vi "실습 5-4 열거형 케이스 선택자.vi"() -> ()   [LabVIEW 2014]
uses:
  <vilib>/measure/NI_MABase.lvlib
panel:
  in  "정지":bool
  in  "열거형":enum16{"사인파", "삼각파", "톱니파", "DC 신호", "노이즈"}(ring)=enum."톱니파"
  out "웨이브폼 그래프":waveform(dbl)(graph)
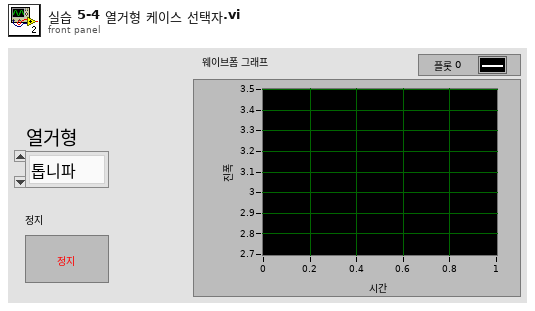
[diagram p1: front panel]
types:
  T1 = enum16{"Sine Wave", "Triangle Wave", "Square Wave", "Sawtooth Wave"}
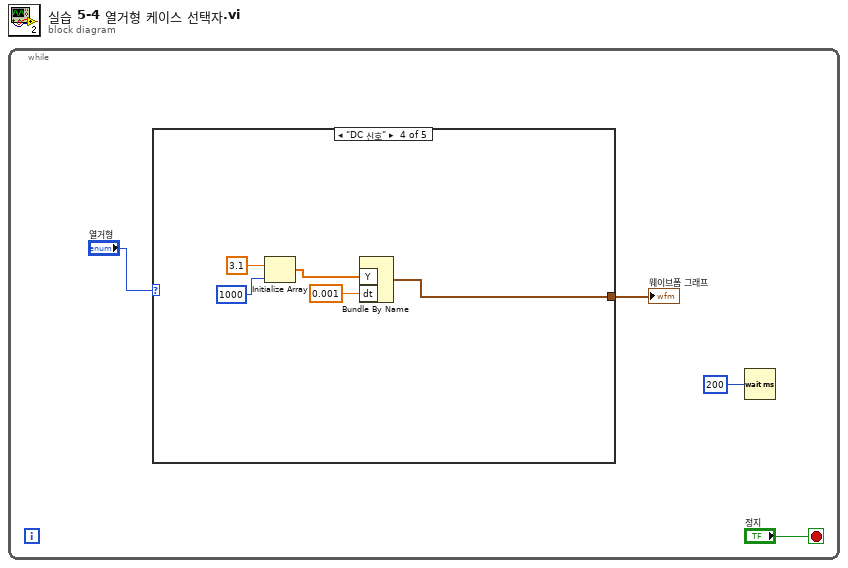
[diagram p0: block diagram]
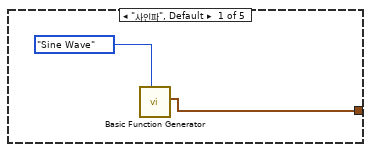
[diagram p2: hidden frame]
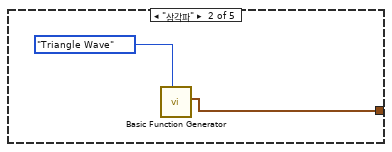
[diagram p3: hidden frame]
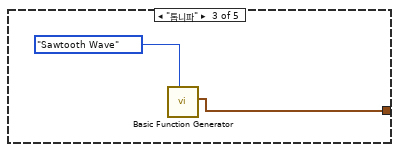
[diagram p4: hidden frame]
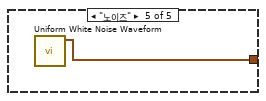
[diagram p5: hidden frame]
diagram:
  n1 = while {
    stop <- "정지" stop-if-true
    n2 = case shown="\"DC 신호\"" "열거형" {
      tunnel: [w5 w7 w9 w12 w16] -> w3
      frame "사인파", Default {
        n3 = call <vilib>:"Basic Function Generator.vi"("signal type"=T1."Sine Wave") -> ("signal out"=w5:waveform(dbl))  [unwired: 8 in, 2 out]
      }
      frame "삼각파" {
        n4 = call <vilib>:"Basic Function Generator.vi"("signal type"=T1."Triangle Wave") -> ("signal out"=w7:waveform(dbl))  [unwired: 8 in, 2 out]
      }
      frame "톱니파" {
        n5 = call <vilib>:"Basic Function Generator.vi"("signal type"=T1."Sawtooth Wave") -> ("signal out"=w9:waveform(dbl))  [unwired: 8 in, 2 out]
      }
      frame "DC 신호" {
        n6 = Initialize Array(3.1 ("원소"), 1000 ("차원 크기")) -> (w13:dbl[])
        n7 = Bundle By Name("Y"=w13, "dt"=0.001) -> (w12:waveform(dbl))  [unwired: 1 in]
      }
      frame "노이즈" {
        n8 = call <vilib>:"Uniform White Noise Waveform.vi"() -> ("signal out"=w16:waveform(dbl))  [unwired: 10 in, 1 out]
      }
    }
    "웨이브폼 그래프" <- w3
    n9 = Wait (ms)(milliseconds to wait=u32 200 ("대기 시간(ms)")) -> ()  [unwired: 1 out]
  }
